vi "Database Connnection Select Data.vi"(7 "condition":string, 8 "error in (no error)":errorcluster caption="错误输入（无错误）", 9 "columns":string[](array[string]), 10 "table":string, 11 "Database Connection 输入":refnum<class "Database Connection.lvclass"> caption="DNL_LabVIEW Object in") -> (0 "error out":errorcluster caption="错误输出", 1 "Data":variant[][](array[variant]), 3 "Database Connection 输出":refnum<class "Database Connection.lvclass"> caption="DNL_LabVIEW Object out")   [LabVIEW 2011, in "Database Connection.lvclass"]
uses:
  Database Connection.lvclass
  Recordset/Database Recordset.lvclass
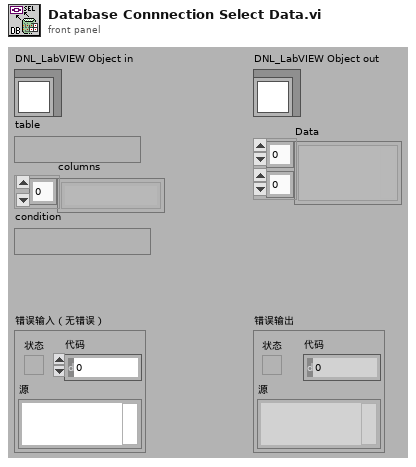
[diagram p1: front panel]
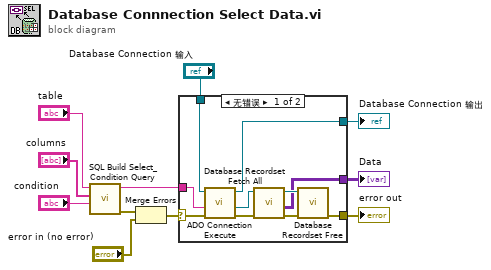
[diagram p0: block diagram]
diagram:
  n1 = call "SQL Build Select_Condition Query.vi"("condition"="condition", "columns"="columns", "table"="table") -> ("error out"=w5:errorcluster, "select query"=w2:string)  [unwired: 7 in]
  n2 = Merge Errors(w5, "error in (no error)") -> (w3:errorcluster)
  n3 = case shown="无错误" w3 {
    selector: w3 -> [w17 w23]
    tunnel: [w14 w23] -> w11
    tunnel: [w12 w22] -> w9
    tunnel: "Database Connection 输入" -> [w21 w22]
    tunnel: w2 -> [w20 _]
    tunnel: [w13 _] -> w1
    frame No Error {
      n4 = call "ADO Connection Execute.vi"("error in (no error)"=w17, "CommandText"=w20, "Database Connection 输入"=w21) -> ("error out"=w18:errorcluster, "Database Recordset输出"=w19:refnum<class "Database Recordset.lvclass">, "Database Connection 输出"=w12:refnum<class "Database Connection.lvclass">)  [unwired: 6 in]
      n5 = call "Database Recordset Fetch All.vi"("error in (no error)"=w18, "Database Recordset 输入"=w19) -> ("error out"=w16:errorcluster, "Data"=w13:variant[][], "Database Recordset 输出"=w15:refnum<class "Database Recordset.lvclass">)  [unwired: 7 in]
      n6 = call "Database Recordset Free.vi"("error in (no error)"=w16, "Database Recordset 输入"=w15) -> ("error out"=w14:errorcluster)  [unwired: 9 in]
    }
    frame Error {
    }
  }
  "error out" <- w11
  "Database Connection 输出" <- w9
  "Data" <- w1
